vi "gyro_analyzer.vi"() -> ()   [LabVIEW 2020]
uses:
  <vilib>/Utility/file.llb/Read Delimited Spreadsheet (string).vi
  <vilib>/Utility/file.llb/Write Delimited Spreadsheet (DBL).vi
panel:
  in  "distance":dbl=1000.0 format="%#_13g"
  in  "Log?":bool
  out "time between timestamps":dbl
  out "distance":dbl
  out "mean speed":dbl
  out "end time":timestamp
  out "auto 1000 m":dbl
  out "manual":dbl
  out "timestamp":dbl
  in  "out file path":path=path "C:/Users/Lenovo/Desktop/1000m_teszt.csv"
  out "distance from manual pos":dbl
  out "XY Graph":cluster{timestamp[], dbl[]}[](graph)
  out "flag-timestamp array":cluster{"String":string, timestamp}[](array[cluster])
  out "time from timestamps":dbl format="%0.3f"
  out "true time from speed":dbl format="%0.3f"
  out "time from manual pos":dbl
  out "mean speed from speed":dbl format="%0.3f"
  out "mean speed from manual pos":dbl format="%0.3f"
  out "header out":T1
  in  "csv file path":path
  out "all rows":string[][](array[string])
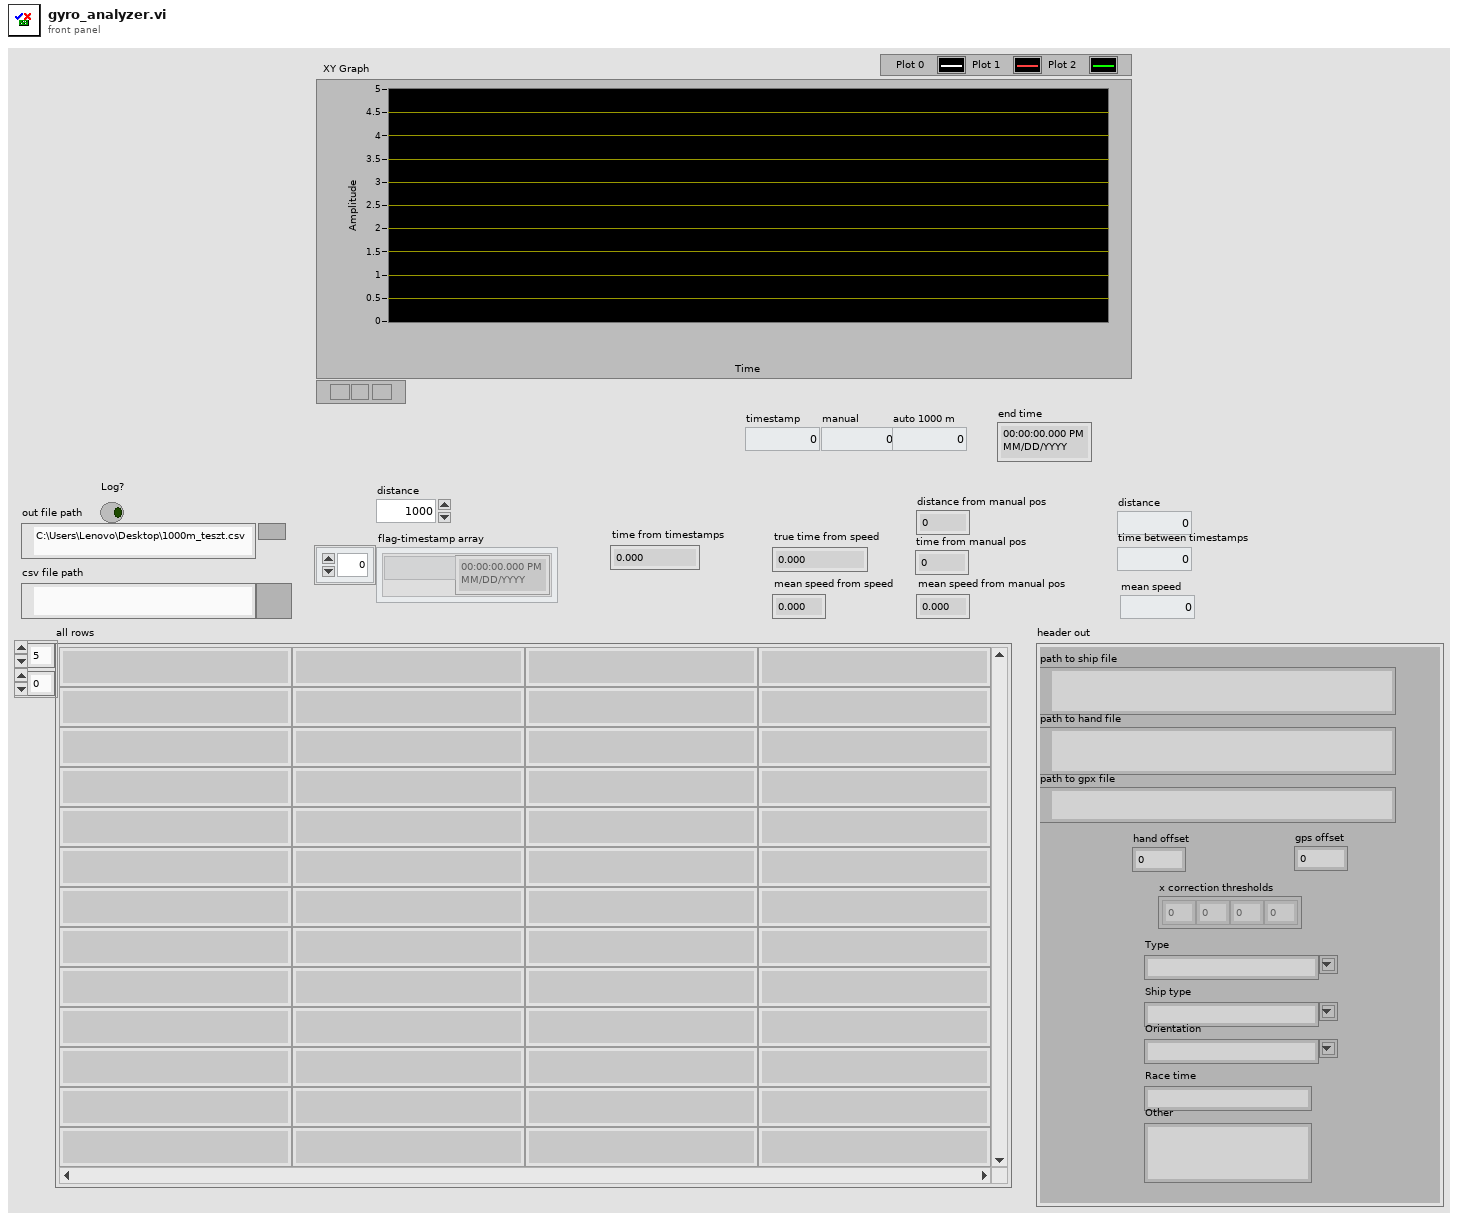
[diagram p1: front panel]
types:
  T1 = cluster{"path to ship file":path, "path to hand file":path, "path to gpx file":path, "hand offset":dbl, "gps offset":dbl, "x correction thresholds":i32[], "Type":string, "Ship type":string, "Orientation":string, "Race time":string, "Other":string}
  T2 = cluster{"Array":timestamp[], "Array":dbl[], "Array":dbl[]}
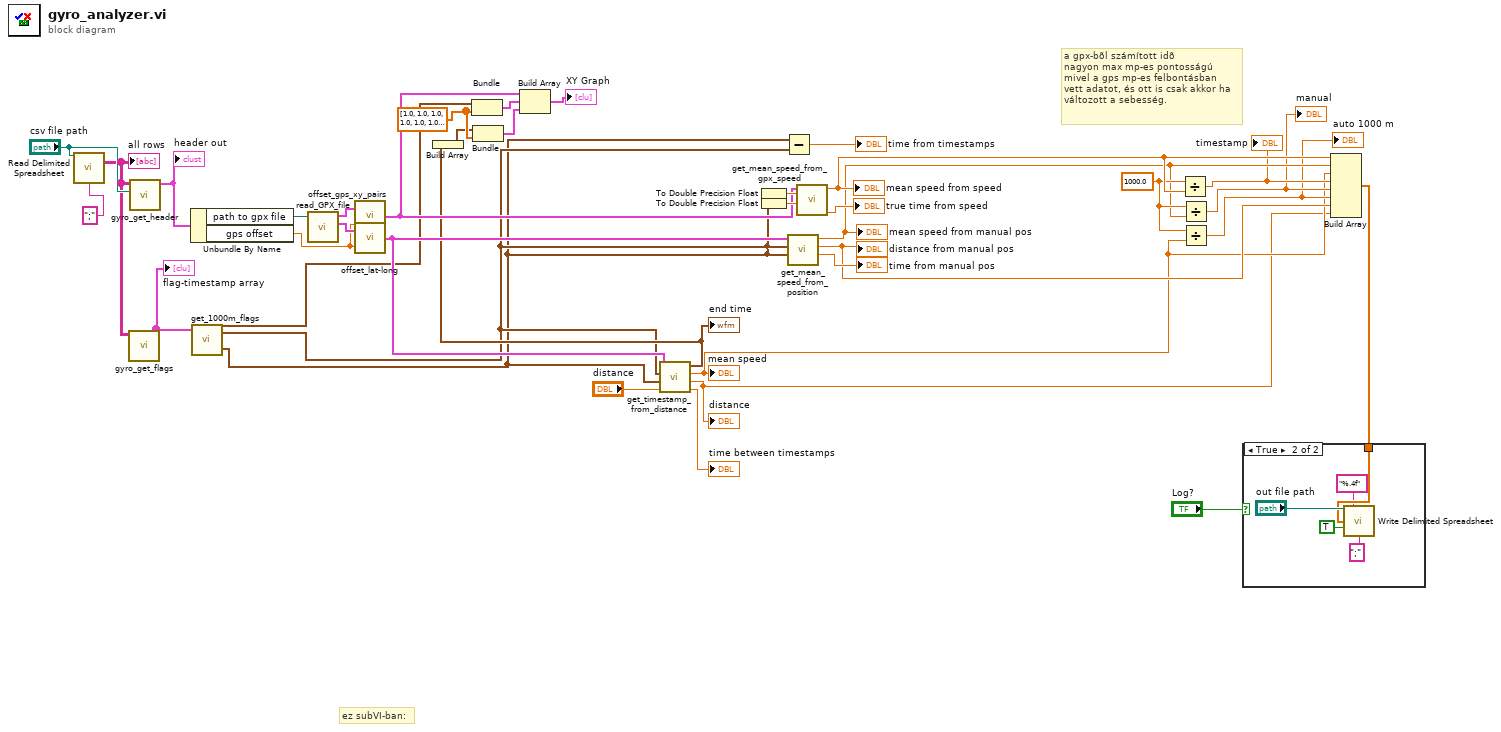
[diagram p0: block diagram]
diagram:
  w19 = 1000.0 ("x")
  w22 = dbl[] [1.0, 1.0, 1.0, 1.0, 1.0, 1.0, 1.0, 1.0, 1.0, 1.0, 1.0, 1.0, 1.0, 1.0, 1.0, 1.0, 1.0, 1.0, 1.0, 1.0]
  # "ez subVI-ban:"
  # "a gpx-bõl számított idõ\nnagyon max mp-es pontosságú\nmivel a gps mp-es felbontásban\nvett adatot, és ott is csak akkor ha\nváltozott a sebesség."
  n1 = call-poly <vilib>:"Read Delimited Spreadsheet.vi"("file path (dialog if empty)"="csv file path", "delimiter (\\t)"=";" ("delimiter (\\t)")) -> ("all rows"=w34:string[][])  [unwired: 8 in, 5 out]
  "all rows" <- w34
  n2 = call "gyro_get_flags.vi"("all rows"=w34) -> ("flag-timestamp array"=w4:cluster{"String":string, timestamp}[])  [unwired: 10 in]
  "flag-timestamp array" <- w4
  n3 = call "gyro_get_header.vi"("csv path"="csv file path", "all rows"=w34) -> ("header out"=w36:T1)  [unwired: 9 in]
  "header out" <- w36
  n4 = Unbundle By Name(w36) -> ("path to gpx file"=w35:path, "gps offset"=w26:dbl)
  n5 = call "get_1000m_flags.vi"("flag-timestamp array"=w4) -> ("1000 m end"=w1:timestamp, "1000 m start"=w2:timestamp, "timestamps"=w3:timestamp[])  [unwired: 2 in]
  n6 = call "read_GPX_file.vi"("GPX File Path"=w35) -> ("lat/lon position"=w33:cluster{timestamp[], dbl[], dbl[]}, "XY Speed data"=w27:cluster{timestamp[], dbl[]})  [unwired: 3 in, 2 out]
  n7 = call "offset_gps_xy_pairs.vi"("offset"=w26, "XY data"=w27) -> ("XY data"=w24:cluster{timestamp[], dbl[]})
  n8 = call "offset_lat-long.vi"("gps offset"=w26, "lat/lon position"=w33) -> ("Cluster"=w13:T2)
  n9 = Bundle("timestamps"=w3, w22) -> (w23:cluster{"timestamps":timestamp[], dbl[]})  [unwired: 1 in]
  n10 = call "get_timestamp_from_distance.vi"("distance"="distance", "manual end"=w1, "start"=w2, "lat/lon position"=w13) -> ("time between timestamps"=→"time between timestamps":dbl, "distance"=w8:dbl, "mean speed"=w9:dbl, "end time"=w5:timestamp)  [unwired: 4 in]
  "end time" <- w5
  "mean speed" <- w9
  "distance" <- w8
  n11 = Build Array(w5) -> (w6:timestamp[])
  n12 = Bundle(w6, w22) -> (w7:cluster{timestamp[], dbl[]})  [unwired: 1 in]
  n13 = Build Array(w24, w23, w7) -> (→"XY Graph":cluster{"timestamps":timestamp[], dbl[]}[])
  n14 = To Double Precision Float(number=w2) -> (double precision float=w28:dbl)
  n15 = To Double Precision Float(number=w1) -> (double precision float=w29:dbl)
  n16 = Subtract(x=w1, y=w2) -> (x-y=→"time from timestamps":dbl)
  n17 = call "get_mean_speed_from_position.vi"("end"=w1, "start"=w2, "lat/lon position"=w13) -> ("dt [s]"=→"time from manual pos":dbl, "distance [m]"=w14:dbl, "mean speed [m/s]"=w18:dbl)  [unwired: 6 in]
  "mean speed from manual pos" <- w18
  "distance from manual pos" <- w14
  n18 = call "get_mean_speed_from_gpx_speed.vi"("to"=w29, "from"=w28, "speed"=w24) -> ("true dt"=→"true time from speed":dbl, "mean"=w20:dbl)  [unwired: 5 in, 2 out]
  "mean speed from speed" <- w20
  n19 = Divide(x=w19, y=w20) -> (x/y=w17:dbl)
  "timestamp" <- w17
  n20 = Divide(x=w19, y=w18) -> (x/y=w16:dbl)
  "manual" <- w16
  n21 = Divide(x=w19, y=w9) -> (x/y=w15:dbl)
  "auto 1000 m" <- w15
  n22 = Build Array(w20, w18, w9, w17, w16, w15, w14, w8) -> (w21:dbl[])
  n23 = case shown="True" "Log?" {
    tunnel: w21 -> [_ w41]
    frame False {
    }
    frame True {
      n24 = call-poly <vilib>:"Write Delimited Spreadsheet.vi"("file path (dialog if empty)"="out file path", "format (%.3f)"="%.4f", "1D data"=w41, "append to file? (new file:F)"=TRUE, "delimiter (\\t)"=";" ("delimiter (\\t)")) -> ()  [unwired: 9 in, 2 out]
    }
  }
